vi "Finish ISTR Cal.vi"(8 "error in (no error)":errorcluster, 9 "Position in":u32, 10 "Cree Comms in":refnum<class "Cree Communications.lvclass">, 11 "Calibration in":refnum<class "Calibration.lvclass">) -> (0 "error out":errorcluster, 1 "Position out":u32, 2 "Cree Comms out":refnum<class "Cree Communications.lvclass">, 3 "Calibration out":refnum<class "Calibration.lvclass">)   [LabVIEW 2015, in "Calibration.lvclass"]
doc: "Turns off the strings not being calibrated. Sets Dim command to 100."
uses:
  Calibration.lvclass
  Classes/Cree Communications/Class/Cree Communications.lvclass
  Classes/Cree Communications/Cree Comms Messages/Write Dim Level/Set Dim Level.lvclass
  Classes/Cree Communications/Cree Comms Messages/Set Current Reference/Set String Current Ref.lvclass
  Classes/Cree Communications/Cree Comms Messages/CC Message/CC Message.lvclass/CC Message.ctl
  Classes/Cree Communications/Cree Comms Messages/CC Message/CC Message.lvclass
  Test Class/Test Class.lvclass
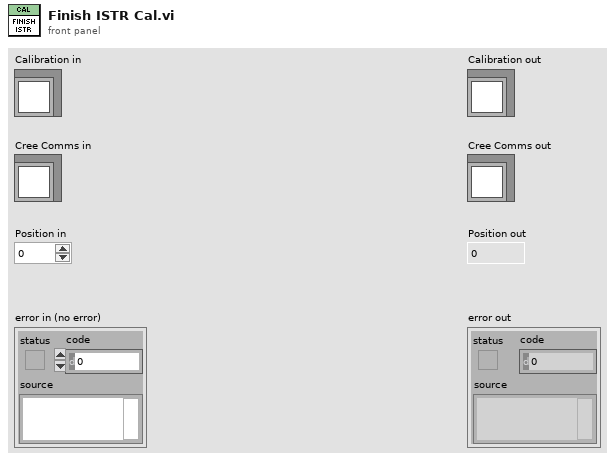
[diagram p1: front panel]
types:
  T1 = cluster{"Current Reference":dbl, "String":enum16{"Red", "BSY1", "BSY2"}}
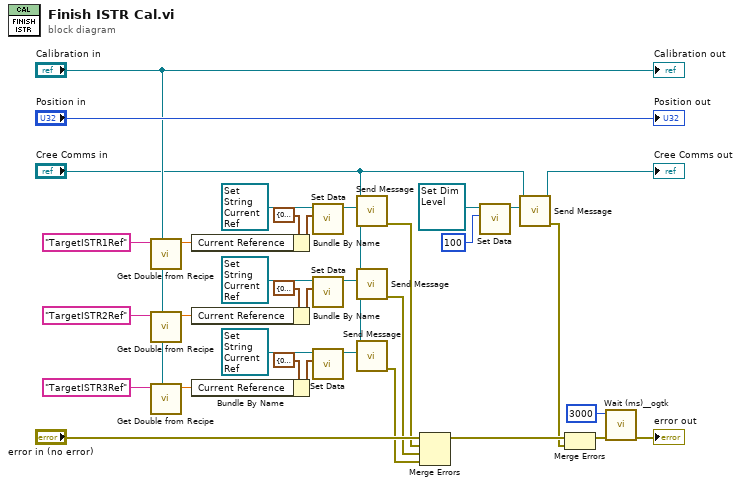
[diagram p0: block diagram]
diagram:
  n1 = call "Get Double from Recipe.vi"("Test Class in"="Calibration in", "Name"="TargetISTR1Ref") -> ("Value"=w22:dbl)  [unwired: 7 in, 2 out]
  n2 = call "Get Double from Recipe.vi"("Test Class in"="Calibration in", "Name"="TargetISTR2Ref") -> ("Value"=w21:dbl)  [unwired: 7 in, 2 out]
  n3 = call "Get Double from Recipe.vi"("Test Class in"="Calibration in", "Name"="TargetISTR3Ref") -> ("Value"=w12:dbl)  [unwired: 7 in, 2 out]
  n4 = Bundle By Name(cluster=T1 {"Current Reference"=0.0, "String"=enum."BSY2"} ("Message Type"), "Current Reference"=w22) -> (w23:T1)
  n5 = Bundle By Name(cluster=T1 {"Current Reference"=0.0, "String"=enum."BSY2"} ("Message Type"), "Current Reference"=w21) -> (w20:T1)
  n6 = Bundle By Name(cluster=T1 {"Current Reference"=0.0, "String"=enum."BSY2"} ("Message Type"), "Current Reference"=w12) -> (w13:T1)
  n7 = call "Set Data.vi"("Data"=w23, "CC Message in"=refnum<class "Set String Current Ref.lvclass"> refnum ("Cree Comms Messages.lvlib:Set String Current Ref.lvclass")) -> ("CC Message out"=w26:refnum<class "Set String Current Ref.lvclass">)  [unwired: 8 in, 1 out]
  n8 = call "Set Data.vi"("Data"=w20, "CC Message in"=refnum<class "Set String Current Ref.lvclass"> refnum ("Cree Comms Messages.lvlib:Set String Current Ref.lvclass")) -> ("CC Message out"=w10:refnum<class "Set String Current Ref.lvclass">)  [unwired: 8 in, 1 out]
  n9 = call "Set Data.vi"("Data"=w13, "CC Message in"=refnum<class "Set String Current Ref.lvclass"> refnum ("Cree Comms Messages.lvlib:Set String Current Ref.lvclass")) -> ("CC Message out"=w9:refnum<class "Set String Current Ref.lvclass">)  [unwired: 8 in, 1 out]
  n10 = call "Send Message.vi"("Cree Comms Message"=w26, "Acrobat Template in"="Cree Comms in") -> ("error out"=w7:errorcluster)  [unwired: 8 in, 1 out]
  n11 = call "Send Message.vi"("Cree Comms Message"=w10, "Acrobat Template in"="Cree Comms in") -> ("error out"=w6:errorcluster)  [unwired: 8 in, 1 out]
  n12 = call "Send Message.vi"("Cree Comms Message"=w9, "Acrobat Template in"="Cree Comms in") -> ("error out"=w8:errorcluster)  [unwired: 8 in, 1 out]
  n13 = Merge Errors("error in (no error)", w7, w6, w8) -> (w3:errorcluster)
  n14 = call "Set Data.vi"("Data"=u8 100 ("Message Type"), "CC Message in"=refnum<class "Set Dim Level.lvclass"> refnum ("Cree Comms Messages.lvlib:Set Dim Level.lvclass")) -> ("CC Message out"=w29:refnum<class "Set Dim Level.lvclass">)  [unwired: 8 in, 1 out]
  n15 = call "Send Message.vi"("Cree Comms Message"=w29, "Acrobat Template in"="Cree Comms in") -> ("error out"=w1:errorcluster, "Acrobat Template out"=→"Cree Comms out":refnum<class "Cree Communications.lvclass">)  [unwired: 8 in]
  n16 = Merge Errors(w3, w1) -> (w2:errorcluster)
  "error out" <- w2
  n17 = call <userlib>:"Wait (ms)__ogtk.vi"("error in (no error)"=w2, "milliseconds to wait"=u32 3000) -> ()  [unwired: 8 in, 2 out]
  "Calibration out" <- "Calibration in"
  "Position out" <- "Position in"
